vi "Event-Image-type.vi"(5 "Menu ref.":refnum<k9>, 7 "Image type":T1, 8 "error in (no error)":errorcluster, 10 "Data ref. in":refnum<data-value>, 11 "UI ref. in":refnum<data-value>) -> (0 "error out":errorcluster, 2 "Data ref.":refnum<data-value>, 3 "UI ref.":refnum<data-value>)   [LabVIEW 2013, in "CameraVision.lvlib" / "CV-UI.lvclass"]
uses:
  CV-UI.lvclass
  Main/CV-Main.lvclass
  Image-selector.ctl
  CV-UI.lvclass/CV-UI.ctl
  Main/Main-actions.ctl
  Read Image.vi
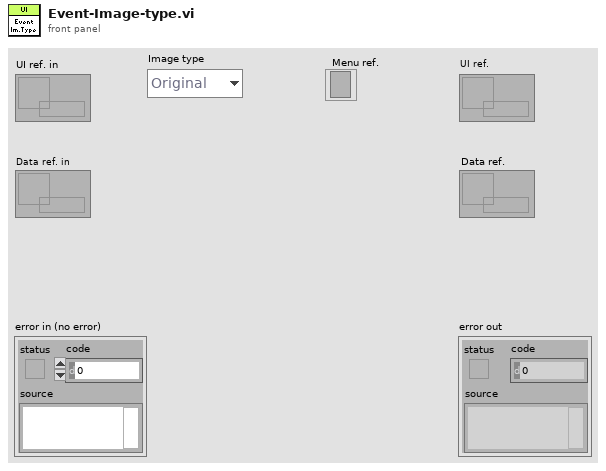
[diagram p1: front panel]
types:
  T1 = typedef "CameraVision.lvlib/CV-UI.lvclass/Image-selector.ctl" = enum16{"Original", "Corrected", "Binary"}
  T2 = typedef "CameraVision.lvlib/CV-Main.lvclass/Main-actions.ctl" = enum16{"Idle", "Initialize", "Load defaults", "Update settings", "Check settings", "Save settings", "Save settings with dialog", "Load settings", "Load data", "Activate", "Start", "Wait for start signal", "Acquire & process", "Iterate", "Stop", "Refresh display", "Refresh status", "View camera settings", "View grabber settings", "Exit"}
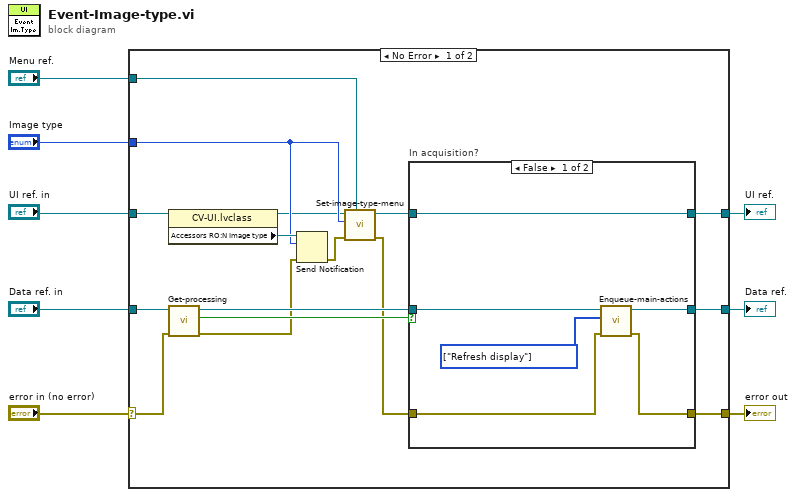
[diagram p0: block diagram]
diagram:
  n1 = case shown="No Error" "error in (no error)" {
    selector: "error in (no error)" -> [w19 w36]
    tunnel: [w18 w36] -> w7
    tunnel: [w21 w35] -> w5
    tunnel: "UI ref. in" -> [w14 w35]
    tunnel: "Data ref. in" -> [w24 w34]
    tunnel: "Image type" -> [w12 _]
    tunnel: [w20 w34] -> w2
    tunnel: "Menu ref." -> [w16 _]
    frame No Error {
      n2 = property class="CV-UI.lvclass"(reference=w14) -> (reference out=w9:refnum<data-value>, "Accessors RO:N Image type"=w13:refnum<notifier>)  [unwired: 1 in, 1 out]
      n3 = call "Get-processing.vi"("error in (no error)"=w19, "Data ref. in"=w24) -> ("error out"=w11:errorcluster, "Processing?"=w22:bool, "Data ref."=w23:refnum<data-value>)  [unwired: 7 in]
      n4 = Send Notification(notification=w12, notifier=w13, error in (no error)=w11) -> (error out=w10:errorcluster)  [unwired: 1 out]
      n5 = call "Set-image-type-menu.vi"("Menu ref."=w16, "error in (no error)"=w10, "Image type"=w12, "UI ref. in"=w9) -> ("error out"=w15:errorcluster, "UI ref."=w17:refnum<data-value>)  [unwired: 6 in]
      n6 = case "In acquisition?" shown="False" w22 {
        tunnel: w17 -> [w28 w32]
        tunnel: w23 -> [w26 w31]
        tunnel: [w28 w32] -> w21
        tunnel: [w25 w31] -> w20
        tunnel: w15 -> [w29 w33]
        tunnel: [w27 w33] -> w18
        frame False {
          w30 = T2[] [enum."Refresh display"] items=["Idle", "Initialize", "Load defaults", "Update settings", "Check settings", "Save settings", "Save settings with dialog", "Load settings", "Load data", "Activate", "Start", "Wait for start signal", "Acquire & process", "Iterate", "Stop", "Refresh display", "Refresh status", "View camera settings", "View grabber settings", "Exit"] ("State array")
          n7 = call "Enqueue-main-actions.vi"("error in (no error)"=w29, "State array"=w30, "Data ref. in"=w26) -> ("error out"=w27:errorcluster, "Data ref."=w25:refnum<data-value>)  [unwired: 6 in, 1 out]
        }
        frame True {
        }
      }
    }
    frame Error {
    }
  }
  "error out" <- w7
  "Data ref." <- w2
  "UI ref." <- w5
